vi "Read Shake Data.vi"(8 "error in (no error)":errorcluster, 11 "Shaker Controller in":refnum<class "Shaker Controller.lvclass">) -> (0 "error out":errorcluster, 3 "Shaker Controller out":refnum<class "Shaker Controller.lvclass">)   [LabVIEW 2020, in "Shaker Controller.lvlib" / "Shaker Controller.lvclass"]
uses:
  Shaker Controller.lvclass
  C:/Program Files (x86)/National Instruments/LabVIEW 2020/vi.lib/ActorFramework/Actor/Actor.lvclass
  <vilib>/ActorFramework/Actor/Actor.lvclass/Actor.ctl
  Shaker Controller.lvclass/Shaker Controller.ctl
  Shaker Controller Interface/Shaker Controller Interface Messages/Report Shake Data Msg/Report Shake Data Msg.lvclass/Report Shake Data Msg.ctl
  <vilib>/ActorFramework/Message Enqueuer/Message Enqueuer.lvclass/Message Enqueuer.ctl
  <vilib>/ActorFramework/Message Enqueuer/Enqueue.vi
  Shaker Controller Interface/Shaker Controller Interface Messages/Report Shake Data Msg/Report Shake Data Msg.lvclass
  C:/Program Files (x86)/National Instruments/LabVIEW 2020/vi.lib/ActorFramework/Message/Message.lvclass
  <vilib>/ActorFramework/Message Priority Queue/Priority Enqueue.vi
  _Abstract Classes/Abstract Shake Monitor/Abstract Shake Monitor.lvclass
  <vilib>/ActorFramework/Actor/Actor.lvclass
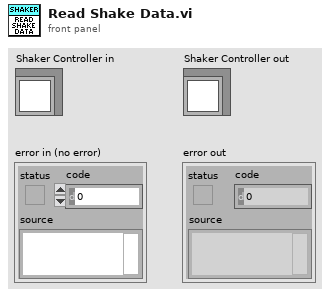
[diagram p1: front panel]
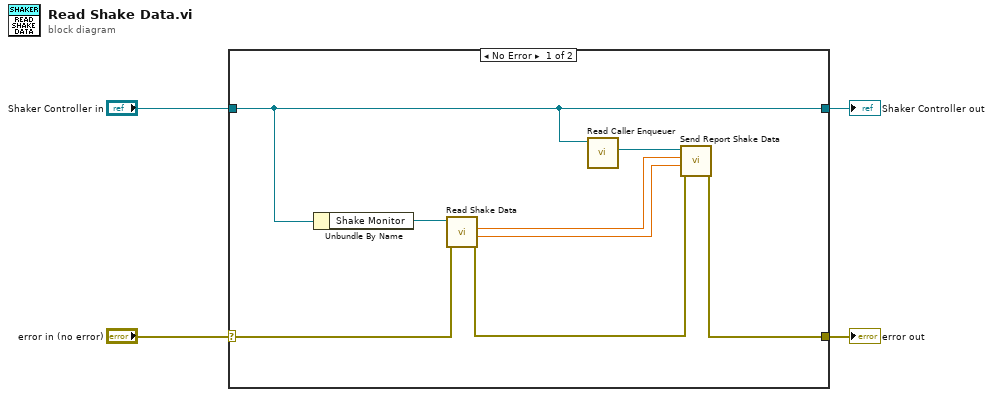
[diagram p0: block diagram]
diagram:
  n1 = case shown="No Error" "error in (no error)" {
    selector: "error in (no error)" -> [w8 w14]
    tunnel: [w10 w14] -> w3
    tunnel: [w12 w13] -> w1
    tunnel: "Shaker Controller in" -> [w12 w13]
    frame No Error {
      n2 = Unbundle By Name(w12) -> ("Shake Monitor"=w9:refnum<class "Abstract Shake Monitor.lvclass">)
      n3 = call-dynamic "Read Shake Data.vi"("error in (no error)"=w8, "Abstract Shake Monitor in"=w9) -> ("error out"=w7:errorcluster, "Shake Amplitude (g)"=w5:dbl, "Shake Frequency (Hz)"=w6:dbl)  [unwired: 6 in, 1 out]
      n4 = call <vilib>:"Read Caller Enqueuer.vi"("Actor"=w12) -> ("Caller Enqueuer"=w11:refnum<class "Message Enqueuer.lvclass">)  [unwired: 10 in]
      n5 = call "Send Report Shake Data.vi"("error in (no error)"=w7, "Amplitude (g)"=w5, "Frequency (Hz)"=w6, "Message Enqueuer"=w11) -> ("error out"=w10:errorcluster)  [unwired: 6 in, 1 out]
    }
    frame Error {
    }
  }
  "error out" <- w3
  "Shaker Controller out" <- w1
